vi "Config Relays.vi"(0 "VISA resource name":refnum<visa-resource-name>, 5 "Relay to Configure (0: Low)":u16(ring) items=["Low", "High"], 7 "Relay Mode (0: Off)":u16(ring) items=["Off", "On", "Alarms", "Zone"], 9 "Channel (1)":i32=1 min=0 max=16 step=1, 11 "error in (no error)":errorcluster, 12 "Alarm Type (0: Low Alarm)":u16(ring) items=["Low Alarm", "High Alarm", "Both Alarms"]) -> (4 "VISA resource name out":refnum<visa-resource-name>, 15 "error out":errorcluster)   [LabVIEW 2012, in "Lake Shore Cryotronics 370.lvlib"]
doc: "This VI configures the parameters of relay control."
uses:
  <instrlib>/Lake Shore Cryotronics 370/Lake Shore Cryotronics 370.lvlib
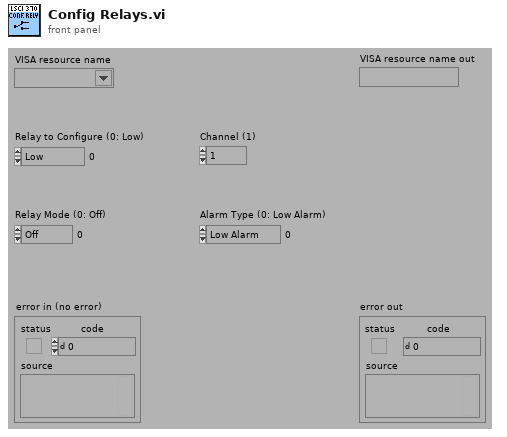
[diagram p1: front panel]
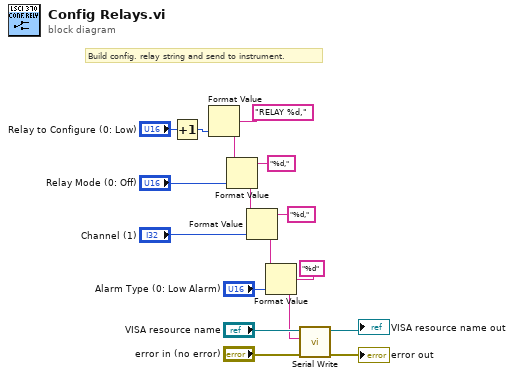
[diagram p0: block diagram]
diagram:
  # "Build config. relay string and send to instrument."
  n1 = Increment(x="Relay to Configure (0: Low)") -> (x+1=w13:u16)
  n2 = Format Value(format string="RELAY %d,", value (0)=w13) -> (output string=w12:string)  [unwired: 1 in]
  n3 = Format Value(string ("")=w12, format string="%d,", value (0)="Relay Mode (0: Off)") -> (output string=w3:string)
  n4 = Format Value(string ("")=w3, format string="%d,", value (0)="Channel (1)") -> (output string=w1:string)
  n5 = Format Value(string ("")=w1, format string="%d", value (0)="Alarm Type (0: Low Alarm)") -> (output string=w6:string)
  n6 = call <instrlib>:"Serial Write.vi"("error in (no error)"="error in (no error)", "Write Buffer (\"\")"=w6, "VISA resource name"="VISA resource name") -> ("error out"=→"error out":errorcluster, "VISA resource name out"=→"VISA resource name out":refnum<visa-resource-name>)  [unwired: 6 in, 1 out]
